vi "dpu_read_str_reg.vi"(5 "raw string? (n)":bool, 7 "byte order (0:big-endian, network order)":T1(ring), 8 "error in":errorcluster, 9 "str len regs (8)":u16=8, 10 "string register":u16, 11 "master":refnum<class "Modbus Master.lvclass">) -> (0 "error out":errorcluster, 2 "string":string, 3 "master out":refnum<class "Modbus Master.lvclass">)   [LabVIEW 2014]
uses:
  protocol/modbus/ni_modbus_api/API/Master/Modbus Master.lvclass
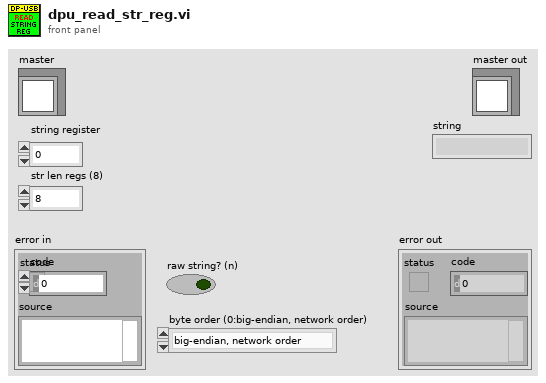
[diagram p1: front panel]
types:
  T1 = enum16{"big-endian, network order", "native, host order", "little-endian"}
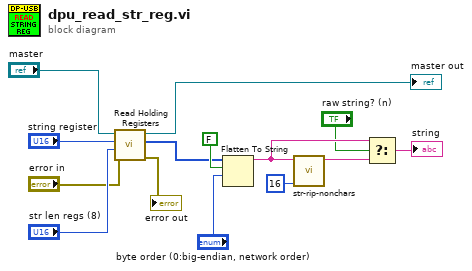
[diagram p0: block diagram]
diagram:
  n1 = call-dynamic "Read Holding Registers.vi"("error in"="error in", "number of inputs"="str len regs (8)", "starting address"="string register", "Modbus master in"="master") -> ("error out"=→"error out":errorcluster, "register values"=w7:u16[], "Modbus master out"=→"master out":refnum<class "Modbus Master.lvclass">)  [unwired: 5 in]
  n2 = Flatten To String(anything=w7, prepend array or string size? (T)=FALSE, byte order (0:big-endian, network order)="byte order (0:big-endian, network order)") -> (data string=w6:string)  [unwired: 1 in, 2 out]
  n3 = call "str-rip-nonchars.vi"("clip string (0=no clipping, pos: clip, neg: clip and stop at first non printable"=16, "String_in"=w6) -> ("String_Out"=w5:string)  [unwired: 9 in]
  n4 = Select(t=w6, s="raw string? (n)", f=w5) -> (s? t:f=→"string":string)
